vi "user32_FindwindowA.vi"(8 "error in (no error)":errorcluster, 10 "lpWindowName":string, 11 "lpClassName":u32) -> (0 "error out":errorcluster, 3 "Return":u32)   [LabVIEW 2020]
uses:
  user32.dll
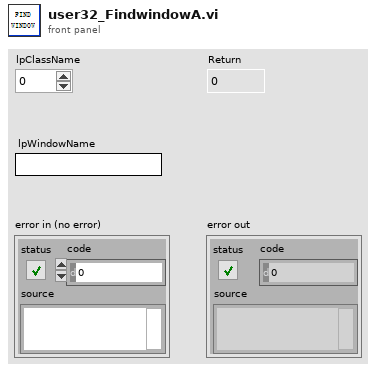
[diagram p1: front panel]
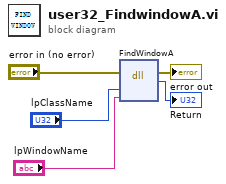
[diagram p0: block diagram]
diagram:
  n1 = dll-call lib="user32.dll" fn="FindWindowA"(error in="error in (no error)", "lpClassName"="lpClassName", "lpWindowName"="lpWindowName") -> (error out=→"error out":errorcluster, "返回值"=→"Return":u32)  [unwired: 4 in, 1 out]
